vi "Get Date String.vi"(8 "error in (no error)":errorcluster, 11 "Barcode Reader in":refnum<class "Barcode Reader.lvclass">) -> (0 "error out":errorcluster, 2 "Date String":string, 3 "Barcode Reader out":refnum<class "Barcode Reader.lvclass">)   [LabVIEW 2020, in "Barcode Reader Second Iteration.lvlib" / "Barcode Reader.lvclass"]
uses:
  Barcode Reader.lvclass
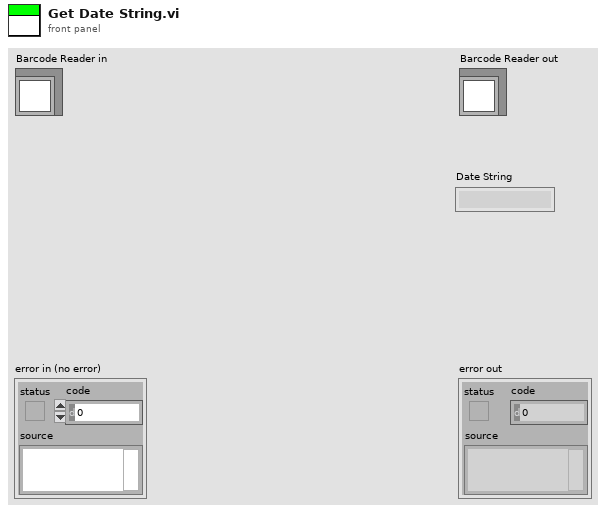
[diagram p1: front panel]
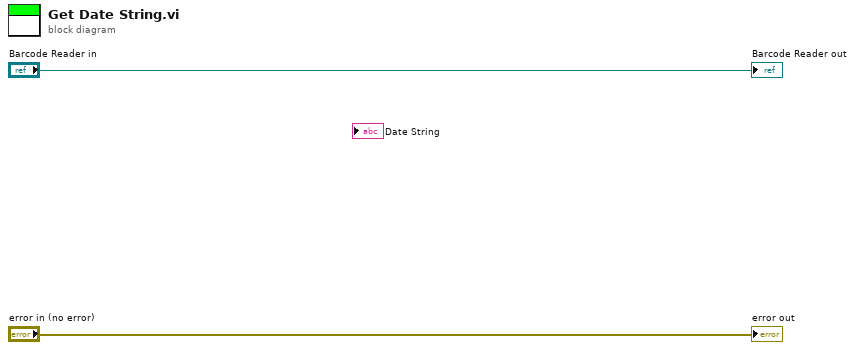
[diagram p0: block diagram]
diagram:
  "error out" <- "error in (no error)"
  "Barcode Reader out" <- "Barcode Reader in"
